vi "GetItemInformationFromProjects.vi"(8 "error in (no error)":errorcluster, 11 "SolutionBuilder in":refnum<class "SolutionBuilder.lvclass">) -> (0 "error out":errorcluster, 3 "SolutionBuilder out":refnum<class "SolutionBuilder.lvclass">)   [LabVIEW 2019, in "SolutionBuilder.lvlib" / "SolutionBuilder.lvclass"]
uses:
  SolutionBuilder.lvclass
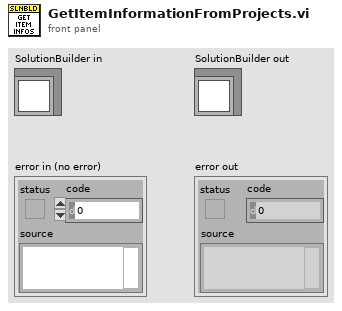
[diagram p1: front panel]
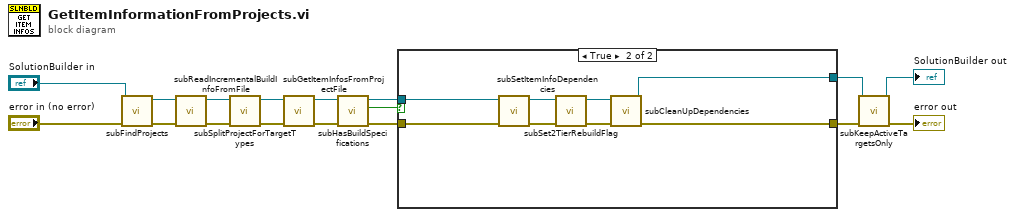
[diagram p0: block diagram]
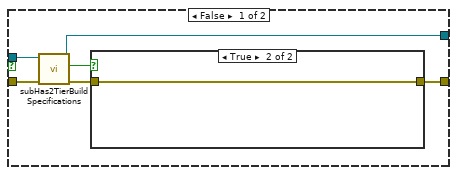
[diagram p2: hidden frame]
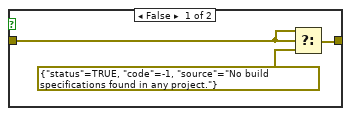
[diagram p3: hidden frame]
diagram:
  n1 = call "subFindProjects.vi"("error in (no error)"="error in (no error)", "SolutionBuilder in"="SolutionBuilder in") -> ("error out"=w9:errorcluster, "SolutionBuilder out"=w10:refnum<class "SolutionBuilder.lvclass">)  [unwired: 8 in]
  n2 = call "subReadIncrementalBuildInfoFromFile.vi"("error in (no error)"=w9, "SolutionBuilder in"=w10) -> ("error out"=w6:errorcluster, "SolutionBuilder out"=w8:refnum<class "SolutionBuilder.lvclass">)  [unwired: 8 in]
  n3 = call "subSplitProjectForTargetTypes.vi"("error in (no error)"=w6, "SolutionBuilder in"=w8) -> ("error out"=w5:errorcluster, "SolutionBuilder out"=w7:refnum<class "SolutionBuilder.lvclass">)  [unwired: 8 in]
  n4 = call "subGetItemInfosFromProjectFile.vi"("error in (no error)"=w5, "SolutionBuilder in"=w7) -> ("error out"=w14:errorcluster, "SolutionBuilder out"=w15:refnum<class "SolutionBuilder.lvclass">)  [unwired: 8 in]
  n5 = call "subHasBuildSpecifications.vi"("error in (no error)"=w14, "SolutionBuilder in"=w15) -> ("error out"=w13:errorcluster, "Has specs?"=w11:bool, "SolutionBuilder out"=w12:refnum<class "SolutionBuilder.lvclass">)  [unwired: 7 in]
  n6 = case shown="True" w11 {
    tunnel: [w20 w35] -> w2
    tunnel: w13 -> [w21 w34]
    tunnel: w12 -> [w22 w33]
    tunnel: [w23 w32] -> w4
    frame False {
      n7 = call "subHas2TierBuildSpecifications.vi"("error in (no error)"=w21, "SolutionBuilder in"=w22) -> ("error out"=w19:errorcluster, "Has specs?"=w18:bool, "SolutionBuilder out"=w20:refnum<class "SolutionBuilder.lvclass">)  [unwired: 7 in]
      n8 = case shown="True" w18 {
        tunnel: w19 -> [w26 w27]
        tunnel: [w25 w27] -> w23
        frame False {
          n9 = Select(t=w26, s=w26, f=errorcluster {"status"=TRUE, "code"=-1, "source"="No build specifications found in any project."} ("t")) -> (s? t:f=w25:errorcluster)
        }
        frame True {
        }
      }
    }
    frame True {
      n10 = call "subSetItemInfoDependencies.vi"("error in (no error)"=w34, "SolutionBuilder in"=w33) -> ("error out"=w29:errorcluster, "SolutionBuilder out"=w31:refnum<class "SolutionBuilder.lvclass">)  [unwired: 8 in]
      n11 = call "subSet2TierRebuildFlag.vi"("error in (no error)"=w29, "SolutionBuilder in"=w31) -> ("error out"=w28:errorcluster, "SolutionBuilder out"=w30:refnum<class "SolutionBuilder.lvclass">)  [unwired: 8 in]
      n12 = call "subCleanUpDependencies.vi"("error in (no error)"=w28, "SolutionBuilder in"=w30) -> ("error out"=w32:errorcluster, "SolutionBuilder out"=w35:refnum<class "SolutionBuilder.lvclass">)  [unwired: 8 in]
    }
  }
  n13 = call "subKeepActiveTargetsOnly.vi"("error in (no error)"=w4, "SolutionBuilder in"=w2) -> ("error out"=→"error out":errorcluster, "SolutionBuilder out"=→"SolutionBuilder out":refnum<class "SolutionBuilder.lvclass">)  [unwired: 8 in]
